vi "write.vi"(11 "Write":T2={"get_vel"=TRUE, "set_vel"=FALSE, "get PID cte"=FALSE, "set PID cte"=FALSE}) -> (3 "s? t:f":T1(ring))   [LabVIEW 2018]
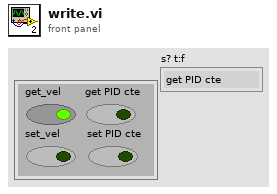
[diagram p1: front panel]
types:
  T1 = enum16{"get PID cte", "Set Vel", "Set PID cte", "get Vel"}
  T2 = cluster{"get_vel":bool, "set_vel":bool, "get PID cte":bool, "set PID cte":bool}
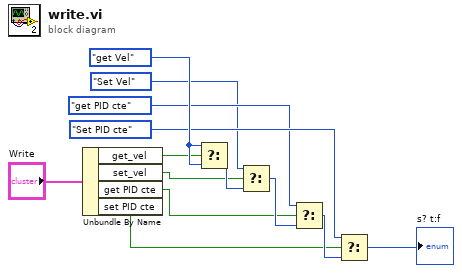
[diagram p0: block diagram]
diagram:
  w12 = T1."get Vel" ("Write")
  n1 = Unbundle By Name("Write") -> ("get_vel"=w2:bool, "set_vel"=w3:bool, "get PID cte"=w4:bool, "set PID cte"=w5:bool)
  n2 = Select(t=w12, s=w2, f=w12) -> (s? t:f=w6:T1)
  n3 = Select(t=T1."Set Vel" ("Write"), s=w3, f=w6) -> (s? t:f=w7:T1)
  n4 = Select(t=T1."get PID cte" ("Write"), s=w4, f=w7) -> (s? t:f=w8:T1)
  n5 = Select(t=T1."Set PID cte" ("Write"), s=w5, f=w8) -> (s? t:f=→"s? t:f":T1)
